vi "set_prr.vi"(8 "error in (no error)":errorcluster, 10 "PRR":sgl, 11 "Laser_Ethernet in":refnum<class "Laser_Ethernet.lvclass">) -> (0 "error out":errorcluster, 3 "Laser_Ethernet out":refnum<class "Laser_Ethernet.lvclass">)   [LabVIEW 2023, in "Laser_Ethernet.lvclass"]
uses:
  Laser_Ethernet.lvclass
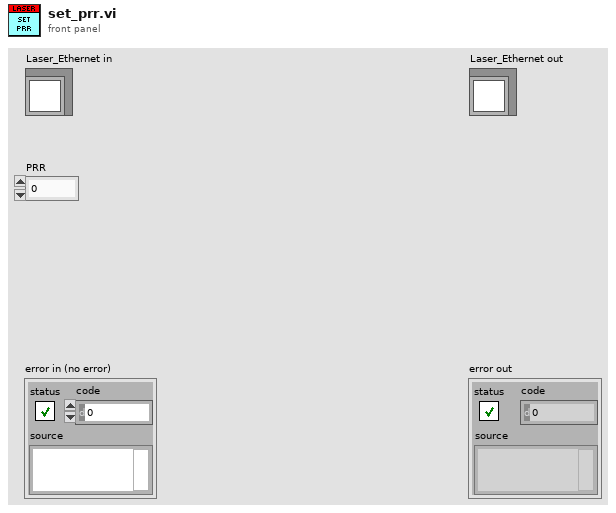
[diagram p1: front panel]
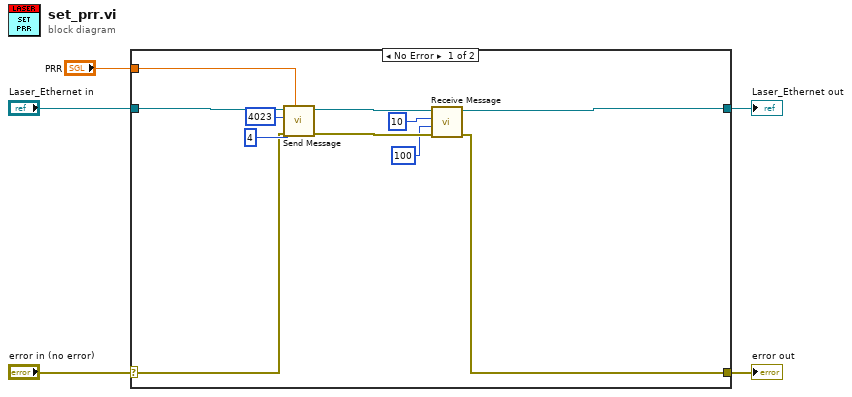
[diagram p0: block diagram]
diagram:
  n1 = case shown="No Error" "error in (no error)" {
    selector: "error in (no error)" -> [w13 w18]
    tunnel: [w8 w18] -> w4
    tunnel: [w10 w17] -> w2
    tunnel: "Laser_Ethernet in" -> [w16 w17]
    tunnel: "PRR" -> [w12 _]
    frame No Error {
      n2 = call "Send Message.vi"("Data"=w12, "error in (no error)"=w13, "Size of Data"=u32 4, "Command"=u16 4023, "object in"=w16) -> ("error out"=w9:errorcluster, "object out"=w11:refnum<class "Laser_Ethernet.lvclass">)  [unwired: 5 in]
      n3 = call "Receive Message.vi"("error in (no error)"=w9, "timeout ms (25000)"=100, "bytes to read"=10, "object in"=w11) -> ("error out"=w8:errorcluster, "object out"=w10:refnum<class "Laser_Ethernet.lvclass">)  [unwired: 5 in, 1 out]
    }
    frame Error {
    }
  }
  "error out" <- w4
  "Laser_Ethernet out" <- w2
